vi "TrajectorySetAbsoluteExecute.vi"(11 "ABSOLUTE EXECUTE":bool) -> ()   [LabVIEW 2023]
uses:
  TrajectoryGlobals.vi
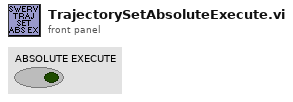
[diagram p1: front panel]
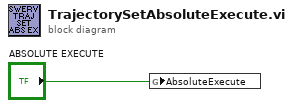
[diagram p0: block diagram]
diagram:
  n1 = global write "TrajectoryGlobals.vi" "AbsoluteExecute"("ABSOLUTE EXECUTE") -> ()
